vi "Set Trigger Level.vi"(8 "error in (no error)":errorcluster, 10 "Trigger Level (1 V)":dbl=1.0 format="%#_4g", 11 "VISA resource name":refnum<visa-resource-name>) -> (0 "error out":errorcluster, 3 "VISA resource name out":refnum<visa-resource-name>)   [LabVIEW 2011, in "SR400.lvlib"]
doc: "TL { v }\nIf v is absent, the TL command returns the gate\ntrigger level. When v is included, the trigger level\nis set to v Volts where -2.000 <= v <= 2.000. The\nresolution is .001 V."
uses:
  SR400.lvlib
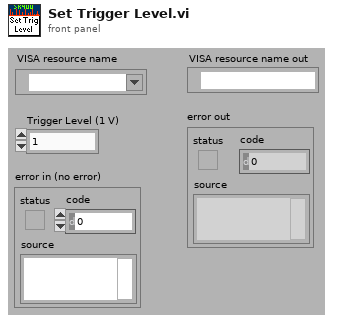
[diagram p1: front panel]
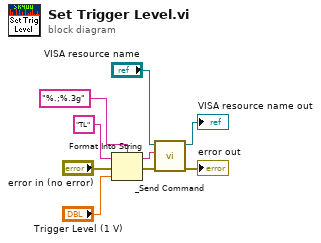
[diagram p0: block diagram]
diagram:
  n1 = Format Into String(format string="%.;%.3g", initial string="TL" ("command"), error in="error in (no error)", "Trigger Level (1 V)") -> (resulting string=w4:string, error out=w3:errorcluster)
  n2 = call "_Send Command.vi"("error in (no error)"=w3, "Command"=w4, "VISA resource name"="VISA resource name") -> ("error out"=→"error out":errorcluster, "VISA resource name out"=→"VISA resource name out":refnum<visa-resource-name>)  [unwired: 1 in, 6 out]
